vi "Get_final_save_path_171213.vi"(2 "Time string":string="Sometimes", 3 "Save directory":path, 4 "File name prefix":string="SavedTrack") -> (0 "File output path":path, 1 "For regions":path)   [LabVIEW 2016]
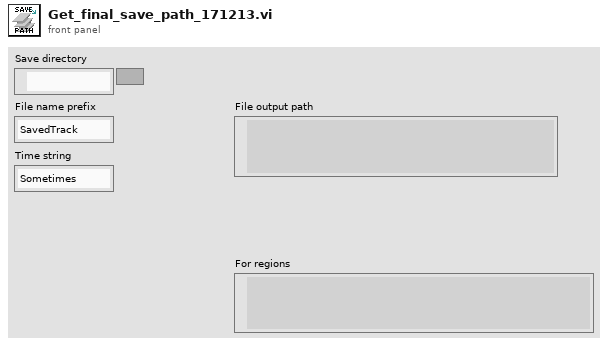
[diagram p1: front panel]
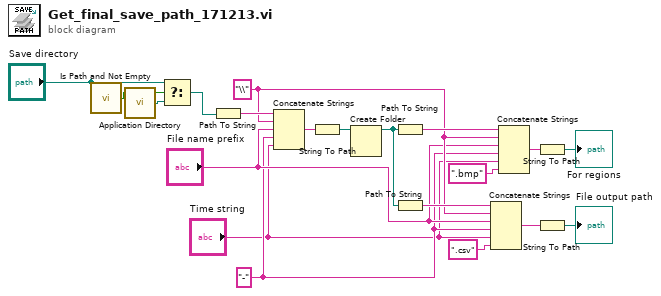
[diagram p0: block diagram]
diagram:
  w4 = "-" ("string")
  w6 = "\\" ("string")
  n1 = call <vilib>:"Is Path and Not Empty.vi"("path"="Save directory") -> ("Is Path and Not Empty?"=w19:bool)  [unwired: 4 in]
  n2 = call <vilib>:"Application Directory.vi"() -> ("Application Directory"=w17:path)
  n3 = Select(t="Save directory", s=w19, f=w17) -> (s? t:f=w20:path)
  n4 = Path To String(path=w20) -> (string=w16:string)
  n5 = Concatenate Strings(w16, w6, "File name prefix", w4, "Time string") -> (w15:string)
  n6 = String To Path(string=w15) -> (path=w14:path)
  n7 = Create Folder(path (use dialog)=w14) -> (created path=w7:path)  [unwired: 2 in, 2 out]
  n8 = Path To String(path=w7) -> (string=w8:string)
  n9 = Path To String(path=w7) -> (string=w13:string)
  n10 = Concatenate Strings(w13, w6, "File name prefix", w4, "Time string", ".csv" ("string")) -> (w12:string)
  n11 = Concatenate Strings(w8, w6, "File name prefix", w4, "Time string", ".bmp" ("string")) -> (w2:string)
  n12 = String To Path(string=w2) -> (path=→"For regions":path)
  n13 = String To Path(string=w12) -> (path=→"File output path":path)
